vi "Renishaw-XL80_GetExpansionCoefficient.vi"(8 "error in (no error)":errorcluster, 11 "Renishaw-XL80 in":refnum<class "Renishaw-XL80.lvclass">) -> (0 "error out":errorcluster, 2 "ExpansionCoefficient":dbl, 3 "Renishaw-XL80 out":refnum<class "Renishaw-XL80.lvclass">)   [LabVIEW 2024, in "Renishaw-XL80.lvclass"]
doc: "Reading this property retrieves the current material expansion coefficient in ppm/°C.\n\nDefinition\nHRESULTget_ExpansionCoefficient( [out, retval] double* pVal);\nParameters\npVal\nA variable that will be set to the current material expansion coefficient (in ppm/°C).\n\nComments\nReading this property will always retrieve the current material expansion coefficient.\n\nThe property will normally return an HRESULT of S_OK. However, it will return E_POINTER if the client supplies a null pointer for pVal."
uses:
  Renishaw-XL80.lvclass
  Renishaw-XL80.lvclass/Renishaw-XL80.ctl
  D:/A.C.M/Example CSharp_64/bin/Debug/Interop.DX10SDKADAPTORLib.dll
  Example CSharp_64/bin/Debug/Interop.DX10SDKADAPTORLib.dll
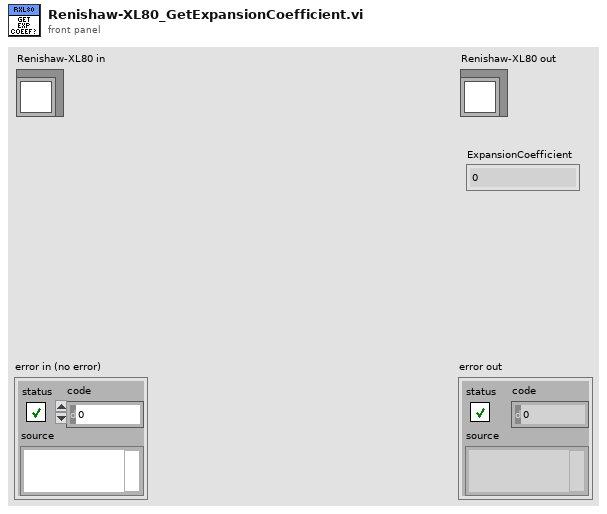
[diagram p1: front panel]
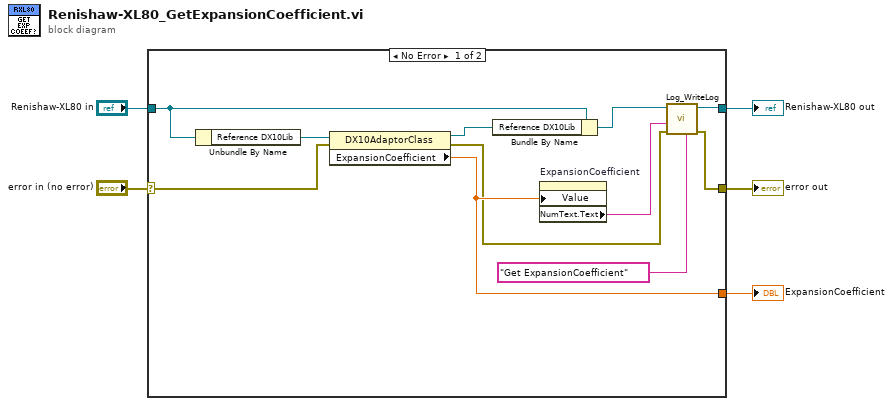
[diagram p0: block diagram]
diagram:
  n1 = case shown="No Error" "error in (no error)" {
    selector: "error in (no error)" -> [w14 w18]
    tunnel: [w8 w18] -> w4
    tunnel: [w10 w17] -> w2
    tunnel: "Renishaw-XL80 in" -> [w13 w17]
    tunnel: [w12 _] -> w1
    frame No Error {
      n2 = Unbundle By Name(w13) -> ("Reference DX10Lib"=w16:refnum<k24>)
      n3 = property class="DX10AdaptorClass"(reference=w16, error in=w14) -> (reference out=w15:refnum<k24>, error out=w6:errorcluster, "ExpansionCoefficient"=w12:dbl)
      n4 = Bundle By Name(cluster=w13, "Reference DX10Lib"=w15) -> (w11:refnum<class "Renishaw-XL80.lvclass">)
      n5 = property on="ExpansionCoefficient" class="DigNum (strict)"("Value"=w12) -> ("NumText.Text"=w9:string)  [unwired: 2 in, 2 out]
      n6 = call-dynamic "Log_WriteLog.vi"("Additional text"="Get ExpansionCoefficient", "error in (no error)"=w6, "Response"=w9, "Log in"=w11) -> ("error out"=w8:errorcluster, "Log out"=w10:refnum<class "Renishaw-XL80.lvclass">)  [unwired: 6 in]
    }
    frame Error {
    }
  }
  "error out" <- w4
  "Renishaw-XL80 out" <- w2
  "ExpansionCoefficient" <- w1
